vi "Open Config File Reference.vi"(8 "error in (no error)":errorcluster, 9 "create file if necessary (T)":bool, 10 "appended path":path, 11 "Configuration File in":refnum<class "Configuration File.lvclass">) -> (0 "error out":errorcluster, 3 "Configuration File out":refnum<class "Configuration File.lvclass">)   [LabVIEW 2019, in "Configuration File.lvlib" / "Configuration File.lvclass"]
doc: "This method takes in a file path to a .ini and opens the reference to it in the class."
uses:
  Configuration File.lvclass
  Configuration File.lvclass/Configuration File.ctl
  <vilib>/Utility/config.llb/NI_LVConfig.lvlib
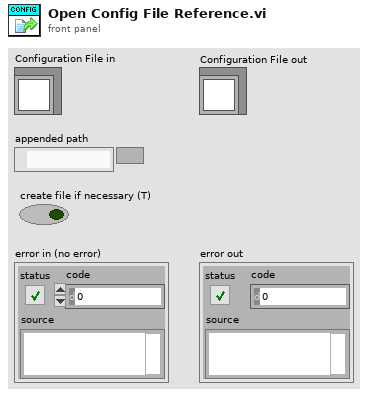
[diagram p1: front panel]
types:
  T1 = typedef "NI_LVConfig.lvlib/Config Data RefNum.ctl" = refnum<k1>
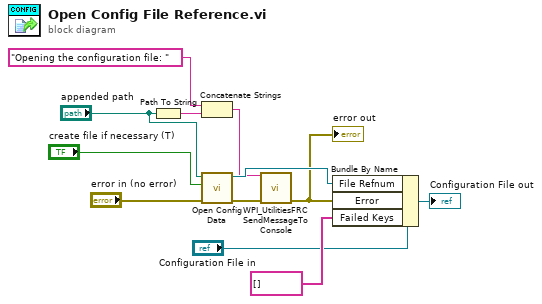
[diagram p0: block diagram]
diagram:
  n1 = Path To String(path="appended path") -> (string=w4:string)
  n2 = Concatenate Strings("Opening the configuration file: " ("string"), w4) -> (w1:string)
  n3 = call <vilib>:"Open Config Data.vi"("error in (no error)"="error in (no error)", "create file if necessary (T)"="create file if necessary (T)", "configuration file path"="appended path") -> ("error out"=w11:errorcluster, "refnum"=w8:T1)  [unwired: 6 in, 1 out]
  n4 = call <vilib>:"WPI_UtilitiesFRC SendMessageToConsole.vi"("Message"=w1, "error in (no error)"=w11) -> ("error out"=w2:errorcluster)  [unwired: 13 in]
  "error out" <- w2
  n5 = Bundle By Name(cluster="Configuration File in", "File Refnum"=w8, "Error"=w2, "Failed Keys"=string[] []) -> (→"Configuration File out":refnum<class "Configuration File.lvclass">)
